vi "DRAFT4.vi"() -> ()   [LabVIEW 2021]
uses:
  <vilib>/Analysis/3filter.llb/Butterworth Filter (DBL).vi
  <vilib>/Analysis/NI_AALBase.lvlib
  <vilib>/ptbypt/NI_PtbyPt.lvlib
panel:
  out "Waveform Graph 7":dynamicdata(graph)
  out "Array Size 2":u32
  out "Array Size":u32
  out "Elapsed time in ms":u32
  in  "stop":bool
  in  "error in (no error)":errorcluster
  out "error out":errorcluster
  in  "loop 1":i32
  out "Waveform Graph 6":dynamicdata(graph)
  out "Waveform Graph 5":dynamicdata(graph)
  out "Waveform Graph 4":dynamicdata(graph)
  out "Waveform Graph 3":dbl[](graph)
  out "Waveform Graph 2":dynamicdata(graph)
  in  "Boolean":bool
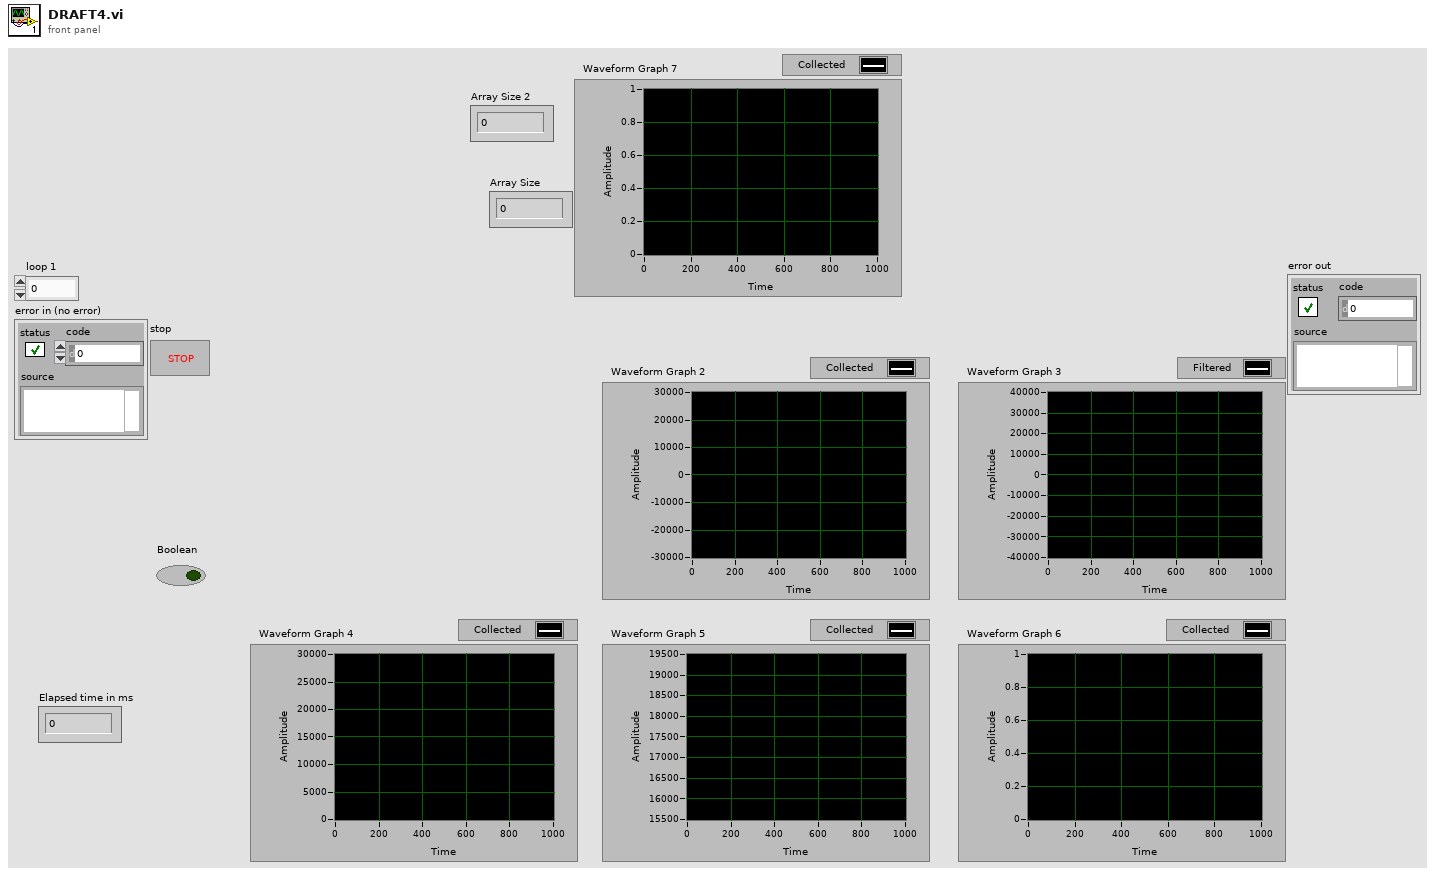
[diagram p1: front panel]
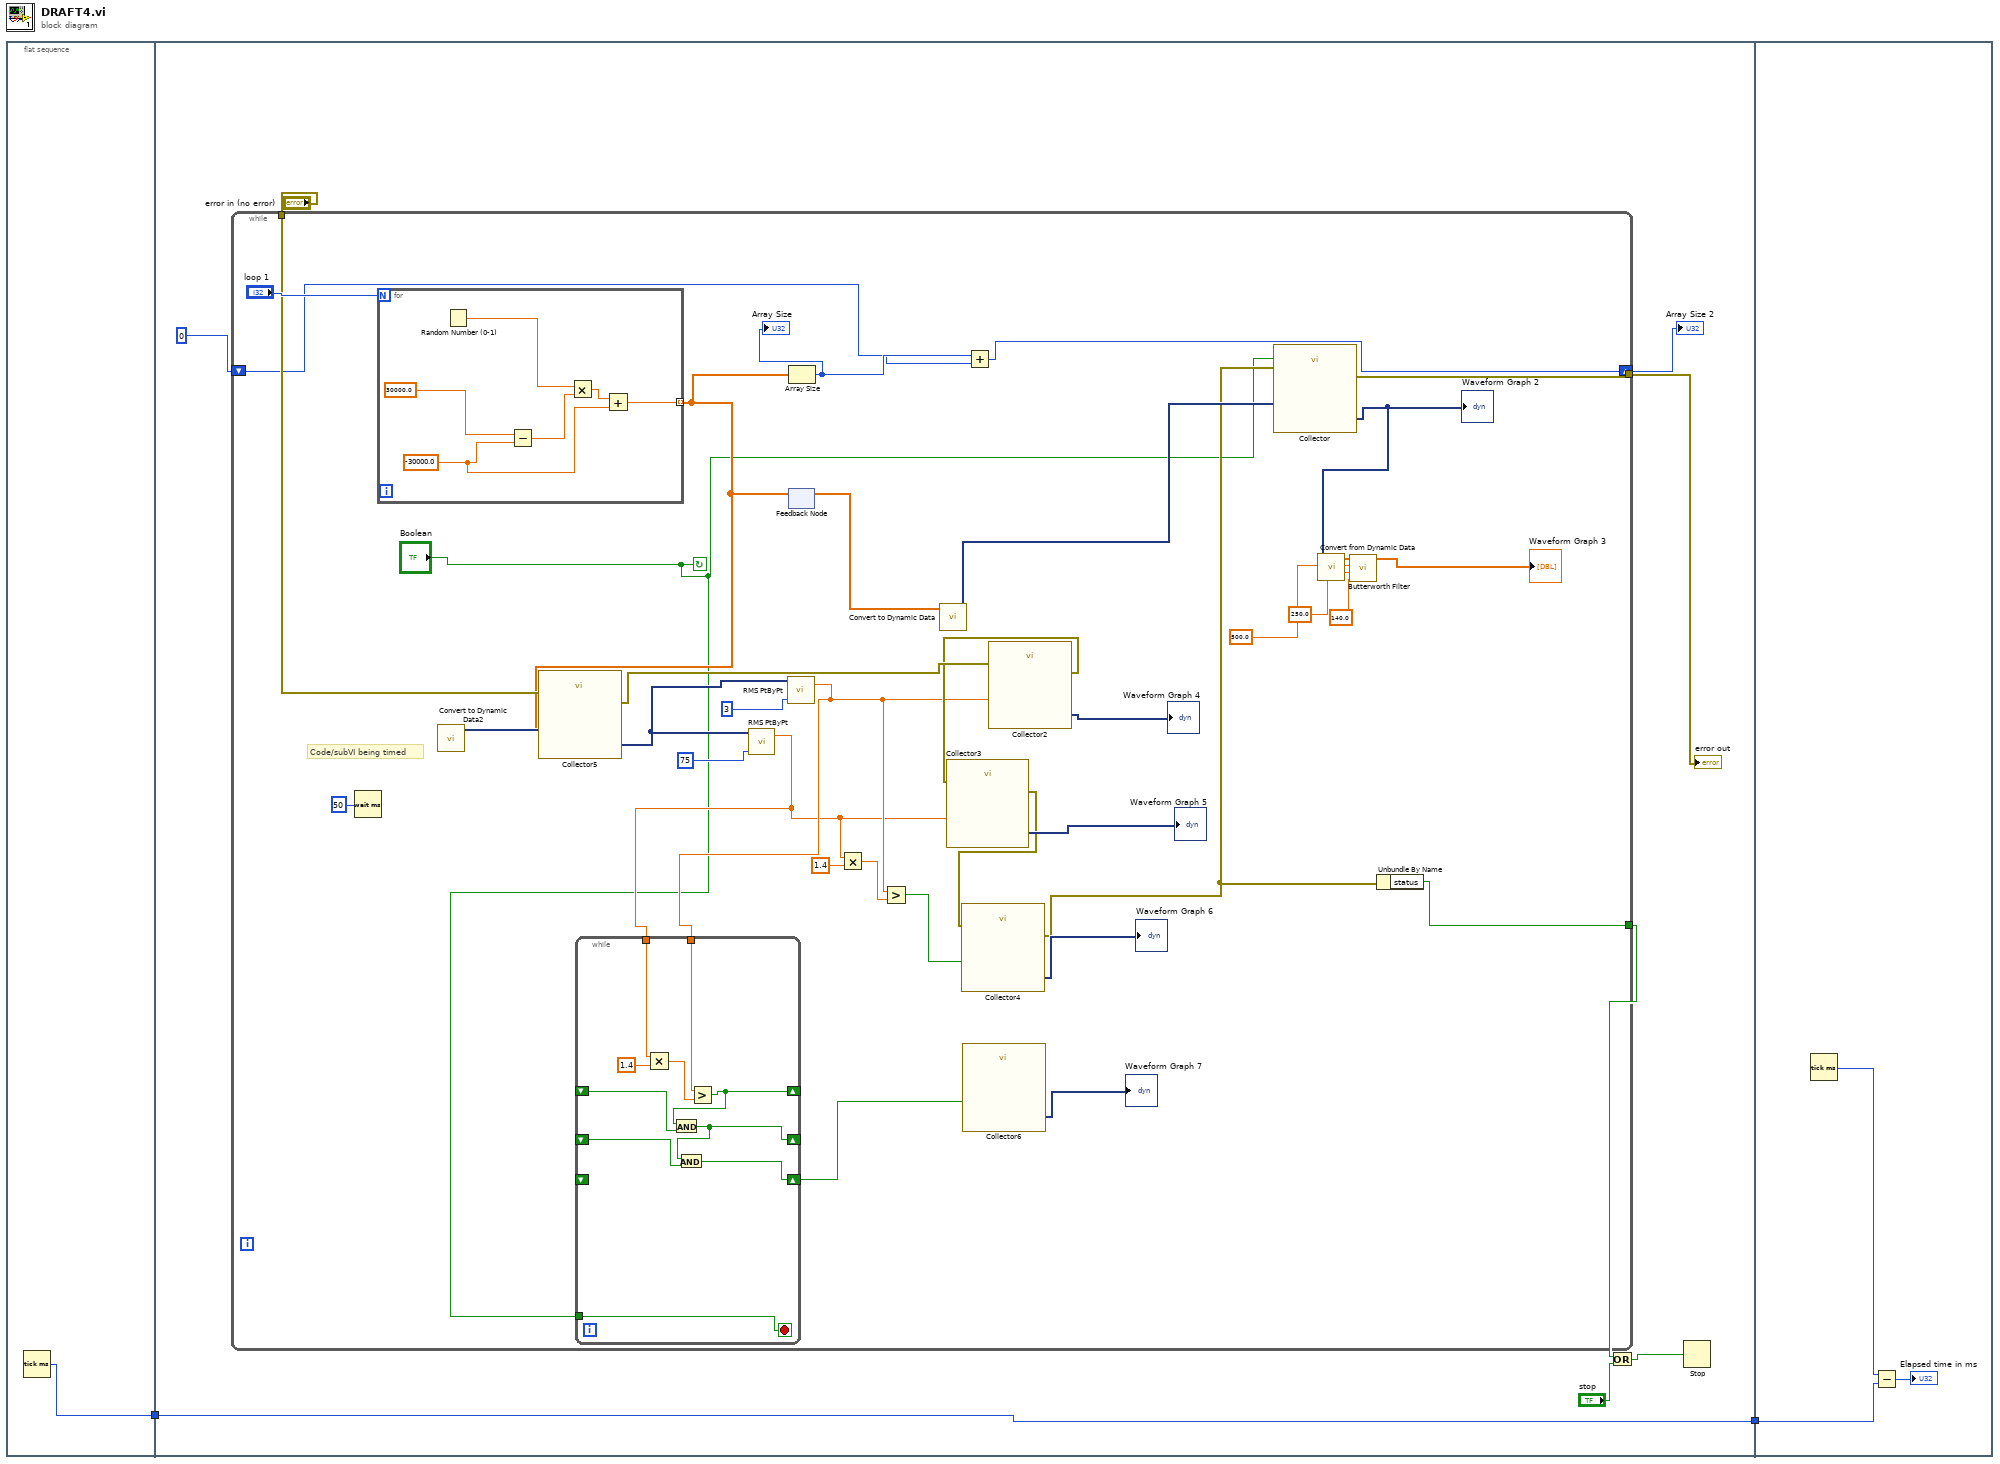
[diagram p0: block diagram]
diagram:
  n1 = flat-sequence {
    tunnel: [w3] -> w2
    tunnel: [w12] -> w1
    tunnel: w2 -> [w12]
    tunnel: w1 -> [w64]
    frame #0 {
      n2 = Tick Count (ms)() -> (millisecond timer value=w3:u32)
    }
    frame #1 {
      # "Code/subVI being timed"
      n3 = while {
        tunnel: "error in (no error)" -> [w29]
        tunnel: [w25] -> w9
        tunnel: [w23] -> w8
        shift-right: [w18] -> w4
        shift-left: 0 -> [w19]
        stop <- "Boolean" continue-if-true
        n4 = for {
          N: "loop 1" -> [_]
          tunnel: [w58] -> w21 mode=indexing
          w60 = -30000.0 ("y")
          n5 = Random Number (0-1)() -> (number: 0 to 1=w59:dbl)
          n6 = Subtract(x=30000.0, y=w60) -> (x-y=w63:dbl)
          n7 = Multiply(x=w59, y=w63) -> (x*y=w62:dbl)
          n8 = Add(x=w62, y=w60) -> (x+y=w58:dbl)
        }
        n9 = call "Convert to Dynamic Data2"("Array"=w21) -> ("Dynamic Data Type"=w31:dynamicdata)  [unwired: 3 in]
        n10 = call "Collector5"("error in (no error)"=w29, "Signals"=w31) -> ("error out"=w28:errorcluster, "Collected Signals"=w30:dynamicdata)  [unwired: 8 in]
        n11 = call <vilib>:"RMS PtByPt.vi"("sample length"=75, "x"=w30) -> ("rms value"=w15:dbl)  [unwired: 2 in, 1 out]
        n12 = call <vilib>:"RMS PtByPt.vi"("sample length"=3, "x"=w30) -> ("rms value"=w16:dbl)  [unwired: 2 in, 1 out]
        n13 = while {
          tunnel: w16 -> [w55]
          tunnel: w15 -> [w54]
          shift-right: [w49] -> _
          shift-left: _ -> [w50]
          shift-right: [w52] -> _
          shift-left: _ -> [w51]
          tunnel: "Boolean" -> [w53]
          shift-right: [w48] -> w13
          shift-left: _ -> [_]
          stop <- w53 stop-if-true
          n14 = Multiply(x=w54, y=1.4) -> (x*y=w56:dbl)
          n15 = Greater?(x=w55, y=w56) -> (0:w52:bool)
          n16 = And(x=w52, y=w51) -> (x .and. y?=w49:bool)
          n17 = And(x=w49, y=w50) -> (x .and. y?=w48:bool)
        }
        n18 = feedback-in #1(w21) -> ()
        n19 = feedback #1() -> (w22:dbl[])  [unwired: 1 in]
        n20 = Array Size(array=w21) -> (size(s)=w20:i32)
        "Array Size" <- w20
        n21 = Multiply(x=w15, y=1.4) -> (x*y=w35:dbl)
        n22 = Greater?(x=w16, y=w35) -> (0:w34:bool)
        n23 = call "Convert to Dynamic Data"("Array"=w22) -> ("Dynamic Data Type"=w39:dynamicdata)  [unwired: 3 in]
        n24 = call "Collector6"("Signals"=w13) -> ("Collected Signals"=→"Waveform Graph 7":dynamicdata)  [unwired: 9 in, 1 out]
        n25 = Add(x=w20, y=w19) -> (x+y=w18:i32)
        n26 = call "Collector2"("error in (no error)"=w28, "Signals"=w16) -> ("error out"=w27:errorcluster, "Collected Signals"=→"Waveform Graph 4":dynamicdata)  [unwired: 8 in]
        n27 = call "Collector3"("error in (no error)"=w27, "Signals"=w15) -> ("error out"=w26:errorcluster, "Collected Signals"=→"Waveform Graph 5":dynamicdata)  [unwired: 8 in]
        n28 = call "Collector4"("error in (no error)"=w26, "Signals"=w34) -> ("error out"=w24:errorcluster, "Collected Signals"=→"Waveform Graph 6":dynamicdata)  [unwired: 8 in]
        n29 = call "Collector"("error in (no error)"=w24, "Enable"="Boolean", "Signals"=w39) -> ("error out"=w25:errorcluster, "Collected Signals"=w42:dynamicdata)  [unwired: 7 in]
        "Waveform Graph 2" <- w42
        n30 = call "Convert from Dynamic Data"("Dynamic Data Type"=w42) -> ("Array"=w44:dbl[])  [unwired: 3 in]
        n31 = call-poly <vilib>:"Butterworth Filter.vi"("low cutoff freq: fl"=140.0, "high cutoff freq: fh"=250.0, "sampling freq: fs"=500.0, "X"=w44) -> ("Filtered X"=→"Waveform Graph 3":dbl[])  [unwired: 4 in, 1 out]
        n32 = Unbundle By Name(w24) -> ("status"=w23:bool)
      }
      "error out" <- w9
      "Array Size 2" <- w4
      n33 = Wait (ms)(milliseconds to wait=u32 50) -> ()  [unwired: 1 out]
      n34 = Or(x=w8, y="stop") -> (x .or. y?=w6:bool)
      n35 = Stop(stop? (T)=w6) -> ()
    }
    frame #2 {
      n36 = Tick Count (ms)() -> (millisecond timer value=w66:u32)
      n37 = Subtract(x=w66, y=w64) -> (x-y=→"Elapsed time in ms":u32)
    }
  }
